vi "ReadAndParsePyFile.vi"(0 "file path (dialog if empty)":path=path "C:/Labview/Projects/WAM_CLK_TEST/support_files/VerifySiTime.py", 11 "error in (no error)":errorcluster) -> (2 "ok?(t)":bool, 3 "regs":string, 6 "Message":string, 15 "error out":errorcluster)   [LabVIEW 2018]
uses:
  <vilib>/Utility/file.llb/Read Delimited Spreadsheet (string).vi
panel:
  out "file path (str)":string
  # "VerifysiTime.py"
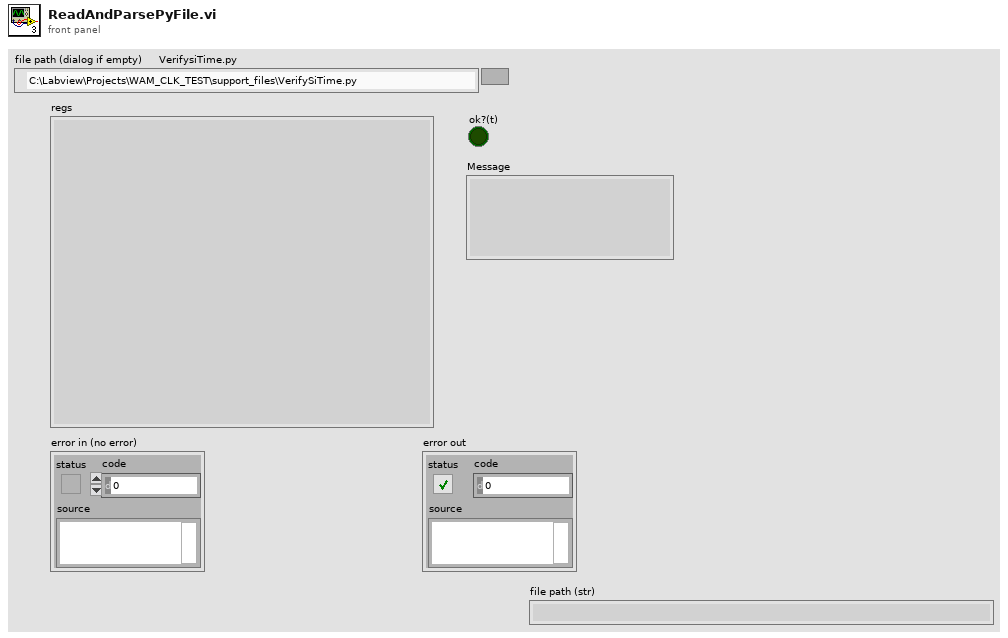
[diagram p1: front panel]
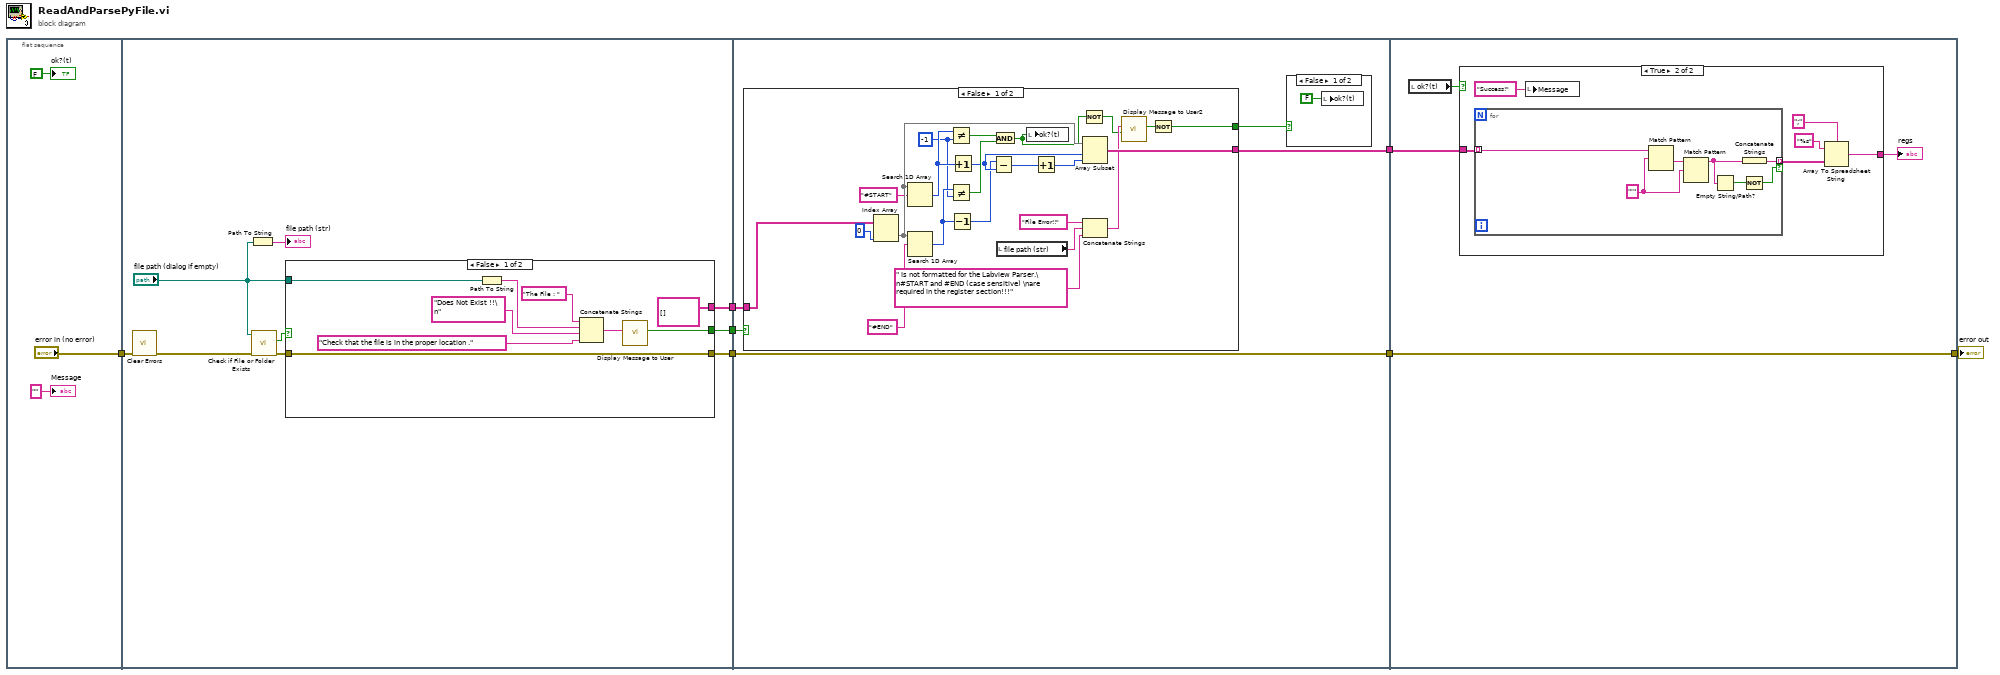
[diagram p0: block diagram]
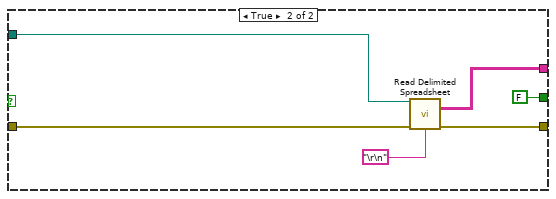
[diagram p2: hidden frame]
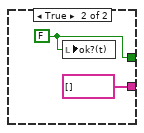
[diagram p4: hidden frame]
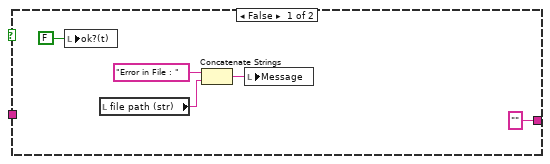
[diagram p5: hidden frame]
diagram:
  n1 = flat-sequence {
    tunnel: ["error in (no error)"] -> w7
    tunnel: w7 -> [w16]
    tunnel: [w19] -> w6
    tunnel: [w15] -> w5
    tunnel: [w11] -> w3
    tunnel: w6 -> [w35]
    tunnel: w5 -> [w38]
    tunnel: [w39] -> w4
    tunnel: w3 -> [w36]
    tunnel: [w36] -> w2
    tunnel: w4 -> [w69]
    tunnel: w2 -> [w66]
    tunnel: [w66] -> w1
    frame #0 {
      "ok?(t)" <- FALSE
      "Message" <- "" ("Message")
    }
    frame #1 {
      n2 = call <vilib>:"Clear Errors.vi"("error in (no error)"=w16) -> ("error out"=w17:errorcluster)  [unwired: 5 in, 1 out]
      n3 = Path To String(path="file path (dialog if empty)") -> (string=→"file path (str)":string)
      n4 = call <vilib>:"Check if File or Folder Exists.vi"("error in (no error)"=w17, "path"="file path (dialog if empty)") -> ("error out"=w12:errorcluster, "file or folder exists?"=w18:bool)  [unwired: 7 in, 1 out]
      n5 = case shown="False" w18 {
        tunnel: [string[][] [] ("all rows") w34] -> w19
        tunnel: "file path (dialog if empty)" -> [w27 w32]
        tunnel: [w22 FALSE ("OK")] -> w15
        tunnel: w12 -> [w20 w30]
        tunnel: [w20 w29] -> w11
        frame False {
          n6 = Path To String(path=w27) -> (string=w21:string)
          n7 = Concatenate Strings("The File : ", w21, "Does Not Exist !!\n" ("string"), "Check that the file is in the proper location ." ("string")) -> (w24:string)
          n8 = call "Display Message to User"("Message"=w24) -> ("OK"=w22:bool)  [unwired: 9 in, 1 out]
        }
        frame True {
          n9 = call-poly <vilib>:"Read Delimited Spreadsheet.vi"("file path (dialog if empty)"=w32, "error in (no error)"=w30, "delimiter (\\t)"="\r\n") -> ("all rows"=w34:string[][], "error out"=w29:errorcluster)  [unwired: 7 in, 4 out]
        }
      }
    }
    frame #2 {
      n10 = case shown="False" w38 {
        tunnel: w35 -> [w51 _]
        tunnel: [w49 string[] []] -> w39
        tunnel: [w41 w64] -> w37
        frame False {
          w54 = -1 ("y")
          n11 = Index Array(array=w51, index (col)=0 ("disabled index (col)")) -> (element=w55:string[])  [unwired: 1 in]
          n12 = Search 1D Array(1D array=w55, element="#START") -> (index of element=w61:i32)  [unwired: 1 in]
          n13 = Search 1D Array(1D array=w55, element="#END") -> (index of element=w60:i32)  [unwired: 1 in]
          n14 = Not Equal?(x=w61, y=w54) -> (x != y?=w62:bool)
          n15 = Not Equal?(x=w60, y=w54) -> (x != y?=w63:bool)
          n16 = Decrement(x=w60) -> (x-1=w56:i32)
          n17 = Increment(x=w61) -> (x+1=w57:i32)
          n18 = Subtract(x=w56, y=w57) -> (x-y=w58:i32)
          n19 = And(x=w62, y=w63) -> (x .and. y?=w44:bool)
          n20 = local read "file path (str)"() -> (w48:string)
          n21 = local write "ok?(t)"(w44) -> ()
          n22 = Increment(x=w58) -> (x+1=w59:i32)
          n23 = Not(x=w44) -> (.not. x?=w43:bool)
          n24 = Array Subset(array=w55, index=w57, length=w59) -> (w49:string[])
          n25 = Concatenate Strings("File Error!!" ("string"), w48, " Is not formatted for the Labview Parser.\n#START and #END (case sensitive) \nare required in the register section!!!" ("string")) -> (w45:string)
          n26 = call "Display Message to User2"("Enable"=w43, "Message"=w45) -> ("OK"=w42:bool)  [unwired: 8 in, 1 out]
          n27 = Not(x=w42) -> (.not. x?=w41:bool)
        }
        frame True {
          w64 = FALSE ("ok?(t)")
          n28 = local write "ok?(t)"(w64) -> ()
        }
      }
      n29 = case shown="False" w37 {
        frame False {
          n30 = local write "ok?(t)"(FALSE ("ok?(t)")) -> ()
        }
        frame True {
        }
      }
    }
    frame #3 {
      n31 = local read "ok?(t)"() -> (w67:bool)
      n32 = case shown="True" w67 {
        tunnel: w69 -> [_ w80]
        tunnel: ["" ("spreadsheet string") w79] -> w68
        frame False {
          n33 = local write "ok?(t)"(FALSE ("ok?(t)")) -> ()
          n34 = local read "file path (str)"() -> (w70:string)
          n35 = Concatenate Strings("Error in File : " ("Message"), w70) -> (w71:string)
          n36 = local write "Message"(w71) -> ()
        }
        frame True {
          n37 = for {
            tunnel: w80 -> [w81] mode=indexing
            tunnel: [w82] -> w77 mode=indexing if=w84
            w86 = "'" ("regular expression")
            n38 = Match Pattern(string=w81, regular expression=w86) -> (after substring=w87:string)  [unwired: 1 in, 3 out]
            n39 = Match Pattern(string=w87, regular expression=w86) -> (before substring=w83:string)  [unwired: 1 in, 3 out]
            n40 = Empty String/Path?(string/path=w83) -> (empty?=w85:bool)
            n41 = Not(x=w85) -> (.not. x?=w84:bool)
            n42 = Concatenate Strings(w83) -> (w82:string)
          }
          n43 = local write "Message"("Success!" ("Message")) -> ()
          n44 = Array To Spreadsheet String(delimiter (Tab)=";", array=w77, 3:"%s" ("format string")) -> (spreadsheet string=w79:string)
        }
      }
      "regs" <- w68
    }
  }
  "error out" <- w1
